vi "Parse XML Comment.vi"(8 "error in (no error)":errorcluster, 9 "Include Inline Comments (F)":bool, 11 "XML Refnum in":refnum<file>) -> (0 "error out":errorcluster, 1 "Comment":string, 3 "XML Refnum out":refnum<file>, 4 "Comment Line Found":bool)   [LabVIEW 2013, in "XML Parser.lvclass"]
uses:
  XML Parser.lvclass
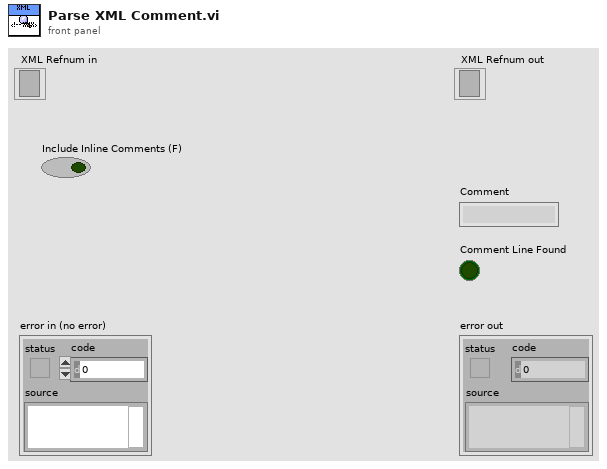
[diagram p1: front panel]
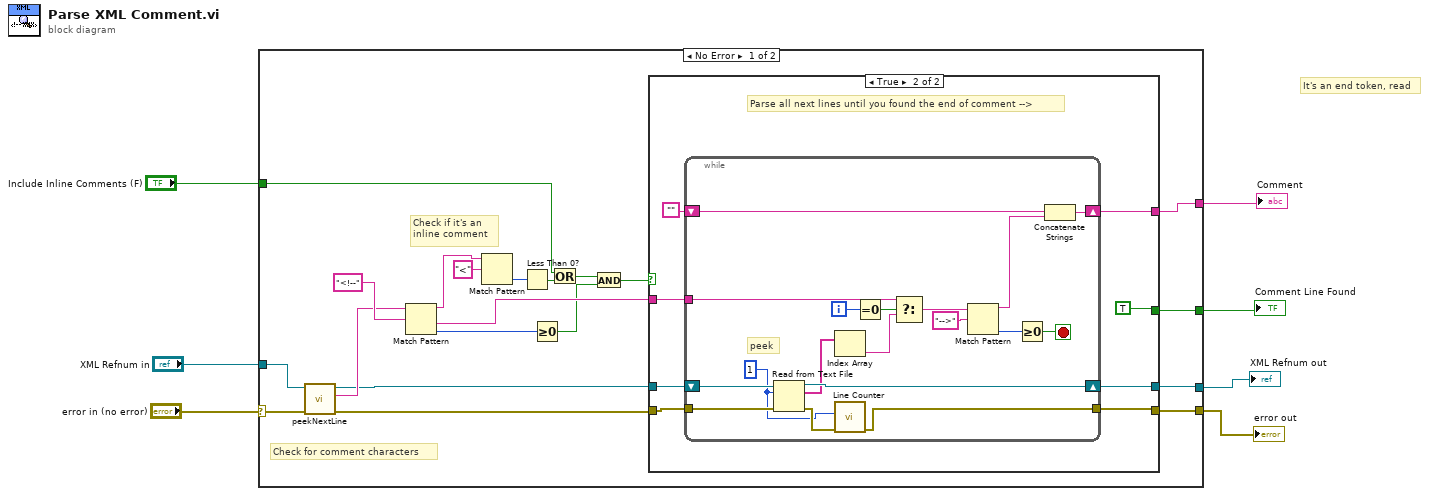
[diagram p0: block diagram]
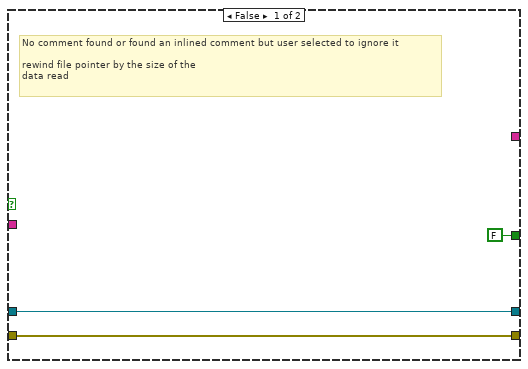
[diagram p2: hidden frame]
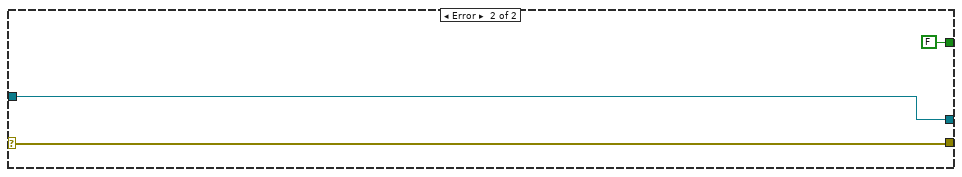
[diagram p3: hidden frame]
diagram:
  # "It's an end token, read"
  n1 = case shown="No Error" "error in (no error)" {
    selector: "error in (no error)" -> [w22 w58]
    tunnel: "XML Refnum in" -> [w20 w59]
    tunnel: [w27 w59] -> w5
    tunnel: [w26 w58] -> w4
    tunnel: [w25 FALSE] -> w3
    tunnel: [w18 _] -> w2
    tunnel: "Include Inline Comments (F)" -> [w10 _]
    frame No Error {
      # "Check if it's an\ninline comment"
      # "Check for comment characters"
      n2 = call "peekNextLine.vi"("error in"=w22, "file* in"=w20) -> ("error out"=w8:errorcluster, "nextLine"=w21:string, "file* out"=w19:refnum<file>)  [unwired: 7 in]
      n3 = Match Pattern(string=w21, regular expression="<!--") -> (before substring=w9:string, after substring=w17:string, offset past match=w23:i32)  [unwired: 1 in, 1 out]
      n4 = Match Pattern(string=w9, regular expression="<") -> (offset past match=w15:i32)  [unwired: 1 in, 3 out]
      n5 = Less Than 0?(x=w15) -> (x < 0?=w12:bool)
      n6 = Greater Or Equal To 0?(x=w23) -> (x >= 0?=w14:bool)
      n7 = Or(x=w10, y=w12) -> (x .or. y?=w13:bool)
      n8 = And(x=w13, y=w14) -> (x .and. y?=w11:bool)
      n9 = case shown="True" w11 {
        tunnel: w19 -> [w29 w37]
        tunnel: w8 -> [w28 w36]
        tunnel: [w29 w33] -> w27
        tunnel: [w28 w34] -> w26
        tunnel: [FALSE TRUE] -> w25
        tunnel: w17 -> [_ w35]
        tunnel: [_ w31] -> w18
        frame False {
          # "No comment found or found an inlined comment but user selected to ignore it\n\nrewind file pointer by the size of the\ndata read"
        }
        frame True {
          # "Parse all next lines until you found the end of comment -->"
          n10 = while {
            shift-right: [w55] -> w31
            shift-left: "" -> [w56]
            tunnel: w36 -> [w53]
            shift-right: [w47] -> w33
            shift-left: w37 -> [w52]
            tunnel: w35 -> [w43]
            tunnel: [w40] -> w34
            i -> [w54]
            stop <- w48 stop-if-true
            w39 = 1 ("count")
            # "peek"
            n11 = Read from Text File(file (use dialog)=w52, count=w39, error in=w53) -> (refnum out=w47:refnum<file>, text=w46:string[], error out=w41:errorcluster)  [unwired: 1 in, 1 out]
            n12 = Index Array(array=w46) -> (element=w44:string)  [unwired: 1 in]
            n13 = call "Line Counter.vi"("error in (no error)"=w41, "# of lines to increment (1)"=w39) -> ("error out"=w40:errorcluster)  [unwired: 8 in, 1 out]
            n14 = Equal To 0?(x=w54) -> (x = 0?=w45:bool)
            n15 = Select(t=w43, s=w45, f=w44) -> (s? t:f=w42:string)
            n16 = Match Pattern(string=w42, regular expression="-->") -> (before substring=w50:string, offset past match=w49:i32)  [unwired: 1 in, 2 out]
            n17 = Greater Or Equal To 0?(x=w49) -> (x >= 0?=w48:bool)
            n18 = Concatenate Strings(w56, w50) -> (w55:string)
          }
        }
      }
    }
    frame Error {
    }
  }
  "XML Refnum out" <- w5
  "error out" <- w4
  "Comment" <- w2
  "Comment Line Found" <- w3
